vi "Translate XBox Data 2.vi"(0 "Steer Axis":i32, 1 "Drive Axis":dbl, 8 "Limit Count Range":dbl=1000000.0, 27 "Disable XBOX?":bool) -> (9 "Filtered Steer Axis":i32, 11 "Steer Counts":dbl, 13 "Filtered Drive Axis":dbl, 15 "Drive Voltage":dbl, 17 "Steer Value Output String":string, 19 "Drive Value Output String":string, 20 "Steer Value Output Number":dbl, 21 "Drive Value Output Number":dbl)   [LabVIEW 2011]
uses:
  <vilib>/express/express arith-compare/Formula/XNode/ExpressFormulaBlockNode.xnode
panel:
  in  "Drive (Keyboard Value)":dbl
  in  "Steer (Keyboard Value)":dbl
  in  "Over ride joystick":bool
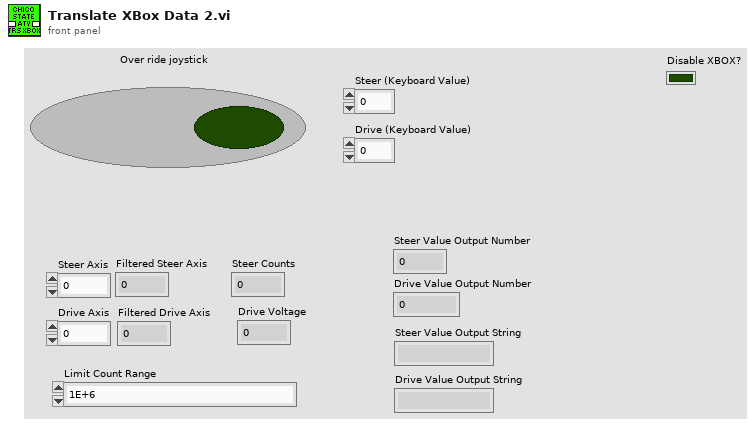
[diagram p1: front panel]
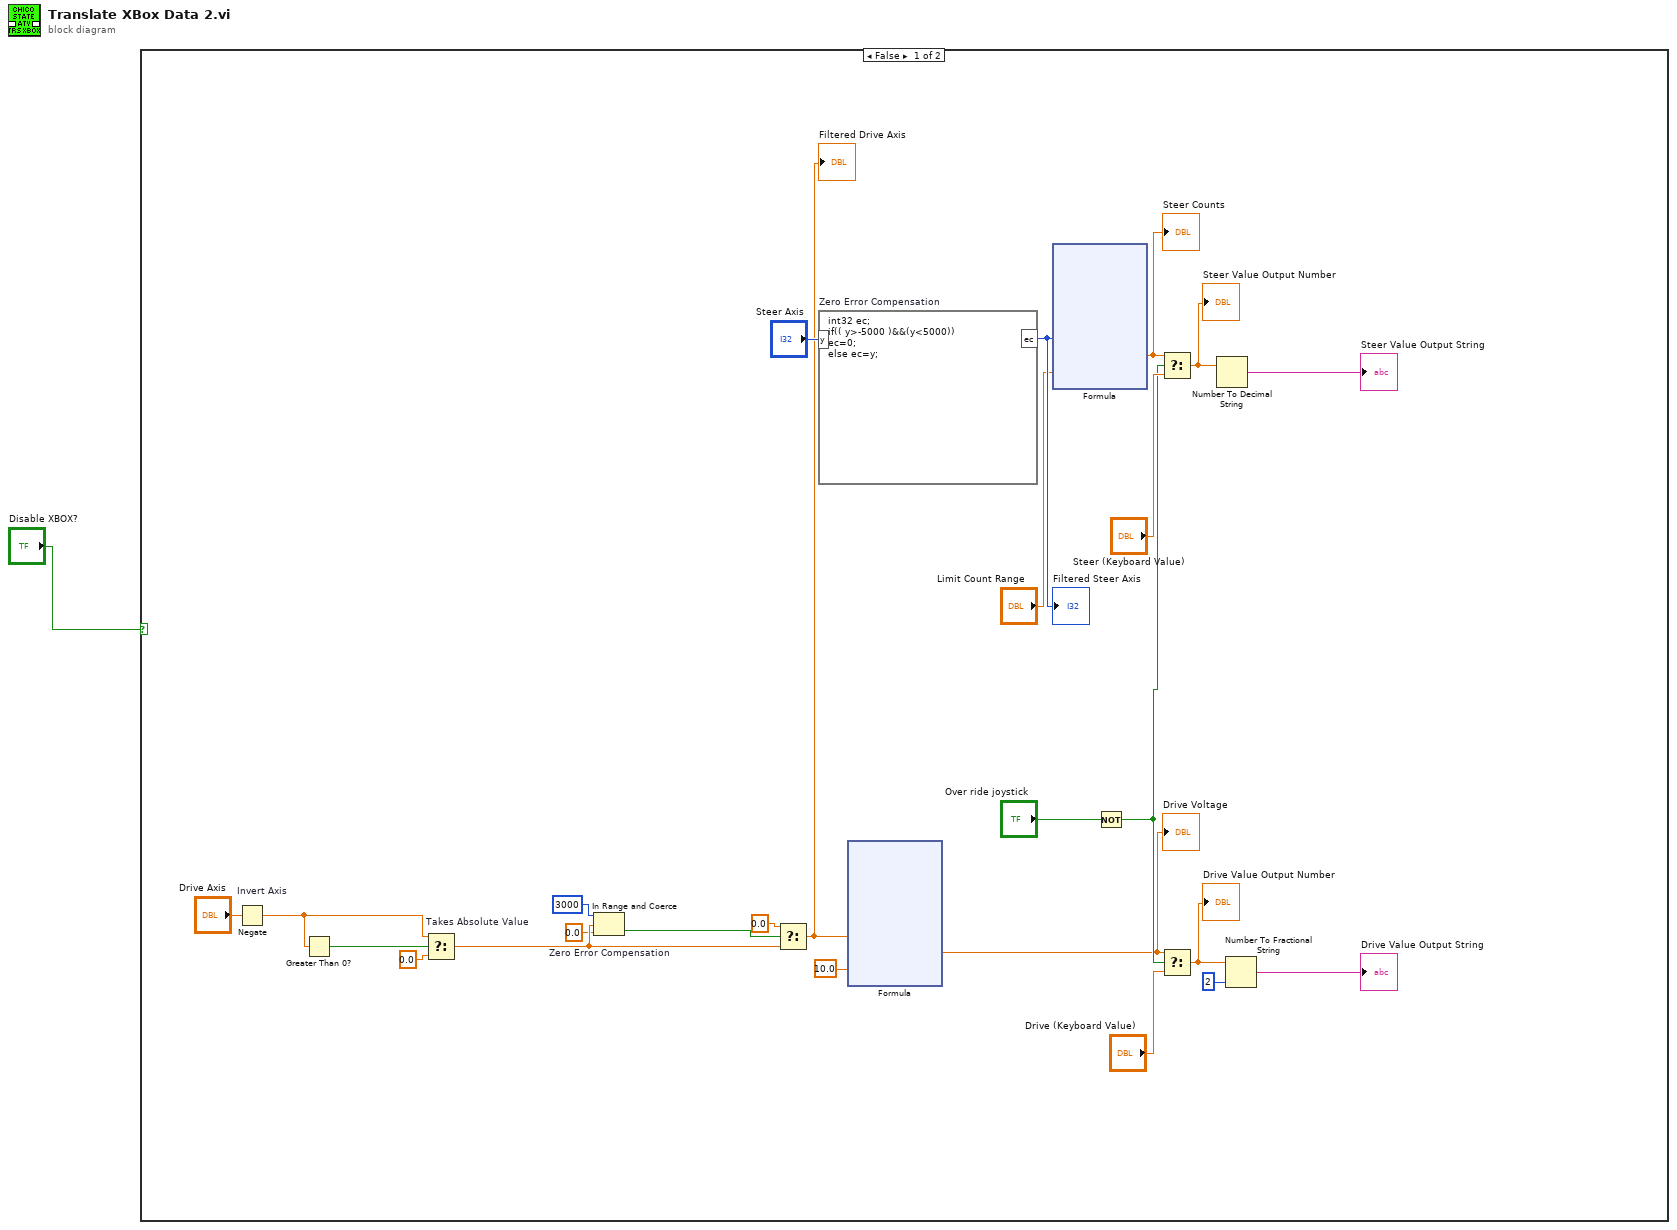
[diagram p0: block diagram]
diagram:
  n1 = case shown="False" "Disable XBOX?" {
    frame False {
      n2 = Negate "Invert Axis"(x="Drive Axis") -> (-x=w25:dbl)
      n3 = Greater Than 0?(x=w25) -> (x > 0?=w26:bool)
      n4 = Select "Takes Absolute Value"(t=w25, s=w26, f=0.0) -> (s? t:f=w22:dbl)
      n5 = In Range and Coerce "Zero Error Compensation"(upper limit=3000, x=w22, lower limit=0.0) -> (In Range?=w23:bool)  [unwired: 1 out]
      n6 = Select(t=0.0, s=w23, f=w22) -> (s? t:f=w8:dbl)
      "Filtered Drive Axis" <- w8
      n7 = formula code="int32 ec;\nif(( y>-5000 )&&(y<5000))\nec=0;\nelse ec=y;" "Zero Error Compensation"("y"="Steer Axis") -> ("ec"=w10:i32)
      "Filtered Steer Axis" <- w10
      n8 = xnode "Formula"("X1"=w8, "X2"=10.0) -> ("Result"=w7:dbl)  [unwired: 1 in, 1 out]
      "Drive Voltage" <- w7
      n9 = xnode "Formula"("X1"=w10, "X2"="Limit Count Range") -> ("Result"=w9:dbl)  [unwired: 1 in, 1 out]
      "Steer Counts" <- w9
      n10 = Not(x="Over ride joystick") -> (.not. x?=w15:bool)
      n11 = Select(t=w9, s=w15, f="Steer (Keyboard Value)") -> (s? t:f=w17:dbl)
      "Steer Value Output Number" <- w17
      n12 = Select(t=w7, s=w15, f="Drive (Keyboard Value)") -> (s? t:f=w18:dbl)
      "Drive Value Output Number" <- w18
      n13 = Number To Decimal String(number=w17) -> (decimal integer string=→"Steer Value Output String":string)  [unwired: 1 in]
      n14 = Number To Fractional String(number=w18, precision (6)=i16 2) -> (F-format string=→"Drive Value Output String":string)  [unwired: 2 in]
    }
    frame True {
    }
  }
